vi "test Get-Set-Get Parameters Configuration File.vi"(8 "error in":errorcluster, 11 "TestCase in":refnum<class "Scripting.lvclass">) -> (0 "error out":errorcluster, 3 "TestCase out":refnum<class "Scripting.lvclass">)   [LabVIEW 2020, in "Scripting.lvclass"]
uses:
  Scripting.lvclass
  Scripting.lvclass/Scripting.ctl
  <vilib>/addons/_JKI Toolkits/VI Tester/TestCase.llb/TestCase.lvclass
  Scripting/Ballard MIL-STD-1553 Scripting.lvlib
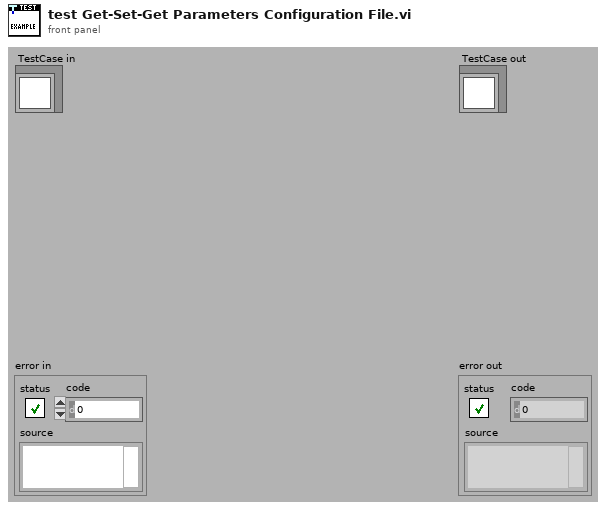
[diagram p1: front panel]
types:
  T1 = cluster{"Hardware File":path, "Parameters File":path}
  T2 = typedef "Custom Device API.lvlib/Custom Device Item Ref.ctl" = u64
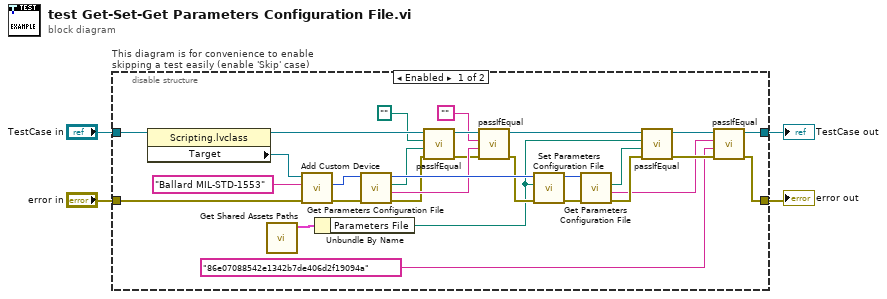
[diagram p0: block diagram]
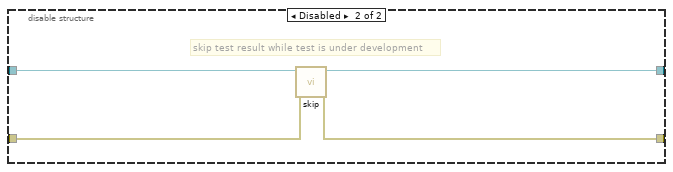
[diagram p2: hidden frame]
diagram:
  n1 = disable-structure "This diagram is for convenience to enable skipping a test easily (enable 'Skip' case)" shown="Enabled" {
    disable-tunnel: "TestCase in" -> [w31 w37]
    disable-tunnel: [w12 w35] -> w1
    disable-tunnel: [w11 w36] -> w3
    disable-tunnel: "error in" -> [w33 w34]
    frame Enabled {
      n2 = property class="Scripting.lvclass"(reference=w31) -> (reference out=w29:refnum<class "Scripting.lvclass">, "Target"=w30:refnum<k24>)  [unwired: 1 in, 1 out]
      n3 = call "Get Shared Assets Paths.vi"() -> ("BC and RTs"=w6:T1)  [unwired: 9 in, 2 out]
      n4 = call "Add Custom Device.vi"("error in"=w33, "name"="Ballard MIL-STD-1553", "target in"=w30) -> ("error out"=w27:errorcluster, "Ballard MIL-STD 1553 custom device"=w28:T2)  [unwired: 6 in, 1 out]
      n5 = Unbundle By Name(w6) -> ("Parameters File"=w5:path)
      n6 = call "Get Parameters Configuration File.vi"("error in"=w27, "Ballard MIL-STD 1553 custom device in"=w28) -> ("error out"=w20:errorcluster, "MD5 checksum"=w21:string, "parameters configuration file"=w23:path, "Ballard MIL-STD 1553 custom device out"=w25:T2)  [unwired: 6 in]
      n7 = call-dynamic "passIfEqual.vi"("error in (no error)"=w20, "y"=w23, "x"=path "", "TestCase in"=w29) -> ("error out"=w18:errorcluster, "TestCase out"=w19:refnum<class "Scripting.lvclass">)  [unwired: 6 in]
      n8 = call-dynamic "passIfEqual.vi"("error in (no error)"=w18, "y"=w21, "x"="", "TestCase in"=w19) -> ("error out"=w17:errorcluster, "TestCase out"=w16:refnum<class "Scripting.lvclass">)  [unwired: 6 in]
      n9 = call "Set Parameters Configuration File.vi"("error in"=w17, "parameters configuration file path"=w5, "Ballard MIL-STD 1553 custom device in"=w25) -> ("error out"=w26:errorcluster, "Ballard MIL-STD 1553 custom device out"=w24:T2)  [unwired: 7 in]
      n10 = call "Get Parameters Configuration File.vi"("error in"=w26, "Ballard MIL-STD 1553 custom device in"=w24) -> ("error out"=w15:errorcluster, "MD5 checksum"=w8:string, "parameters configuration file"=w10:path)  [unwired: 6 in, 1 out]
      n11 = call-dynamic "passIfEqual.vi"("error in (no error)"=w15, "y"=w10, "x"=w5, "TestCase in"=w16) -> ("error out"=w14:errorcluster, "TestCase out"=w13:refnum<class "Scripting.lvclass">)  [unwired: 6 in]
      n12 = call-dynamic "passIfEqual.vi"("error in (no error)"=w14, "y"="86e07088542e1342b7de406d2f19094a" ("MD5 checksum"), "x"=w8, "TestCase in"=w13) -> ("error out"=w11:errorcluster, "TestCase out"=w12:refnum<class "Scripting.lvclass">)  [unwired: 6 in]
    }
    frame Disabled {
      # "skip test result while test is under development"
      n13 = call <vilib>:"skip.vi"("error in (no error)"=w34, "TestCase in"=w37) -> ("error out"=w36:errorcluster, "TestCase out"=w35:refnum<class "Scripting.lvclass">)  [unwired: 8 in]
    }
  }
  "error out" <- w3
  "TestCase out" <- w1
